vi "Precharge Control.vi"() -> ()   [LabVIEW 2014]
uses:
  Shutdown State Machine.lvsc/State.ctl
  Shutdown State Machine.lvsc/Inputs.ctl
  Shutdown State Machine.lvsc/StatechartState.ctl
  Shutdown State Machine.lvsc/CompanionDiagram.vi/2/SC Main.vi
  Shutdown State Machine.lvsc/CompanionDiagram.vi/2/Upd State.vi
  Shutdown State Machine.lvsc/CompanionDiagram.vi/2/Trans Graph0.vi
  Shutdown State Machine.lvsc/CompanionDiagram.vi/2/EnterGraphCore.vi
  <vilib>/FPGAPlugInAG/sbRIO-9626/niLvFpga_Open_sbRIO-9626.vi
  <vilib>/rvi/interface/common/dynamic/niFpgaDynamicAddResources.vi
  Global Data.vi
  <vilib>/Utility/error.llb/Error Cluster From Error Code.vi
  <vilib>/rvi/errors/niLvFpgaAdjustHostInterfaceError.vi
  Shutdown State Machine.lvsc/CompanionDiagram.vi
  <vilib>/FPGAPlugInAG/Dynamic/niLvFpga_Close_Dynamic.vi
  <vilib>/rvi/interface/nirviOpenFPGA/nirviOpenFPGA.xnode
  FPGA Bitfiles/FormulaElectric2_FPGATarget_FPGA_8a5J0mMac2U.lvbitx
  FPGA/Sensor Library/FPGA.vi
  Shutdown State Machine.lvsc/Trigger.ctl
  <vilib>/rvi/interface/nirviReadWriteControl/nirviReadWriteControl.xnode
  <vilib>/Statechart/Infrastructure/RTStatechart/RunTime SCN.xnode
  Shutdown State Machine.lvsc/Outputs.ctl
  AIR Status.ctl
  Shutdown State Machine.lvsc
  <vilib>/rvi/interface/nirviCloseFPGA/nirviCloseFPGA.xnode
  <vilib>/rvi/interface/Simulation/niFpgaSimulationCallBeginRW.vi
  NiFpgaLv.dll
panel:
  out "Shutdown State":T1
  in  "Precharge Time (msec)":u32=4000
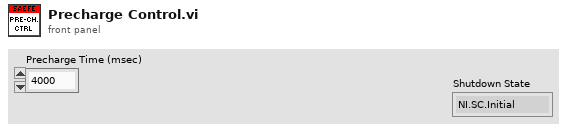
[diagram p1: front panel]
types:
  T1 = typedef "Shutdown State Machine.lvsc/State.ctl" = enum16{"NI.SC.Initial", "NI.SC.History", "NI.SC.ShallowHistory", "NI.SC.Terminal", "Precharge Finished/AIRs On", "Precharge", "TSMS Off"}
  T2 = typedef "Shutdown State Machine.lvsc/Inputs.ctl" = cluster{"TSMS Status In":bool, "Precharge Time":u32}
  T3 = typedef "Shutdown State Machine.lvsc/Outputs.ctl" = cluster{"Positive AIR Enable":bool, "AIR Status":T4, "Coolant Pump":bool}
  T4 = typedef "AIR Status.ctl" = enum16{"Off", "Precharge", "On"}
  T5 = typedef "Shutdown State Machine.lvsc/StatechartState.ctl" = T1[]
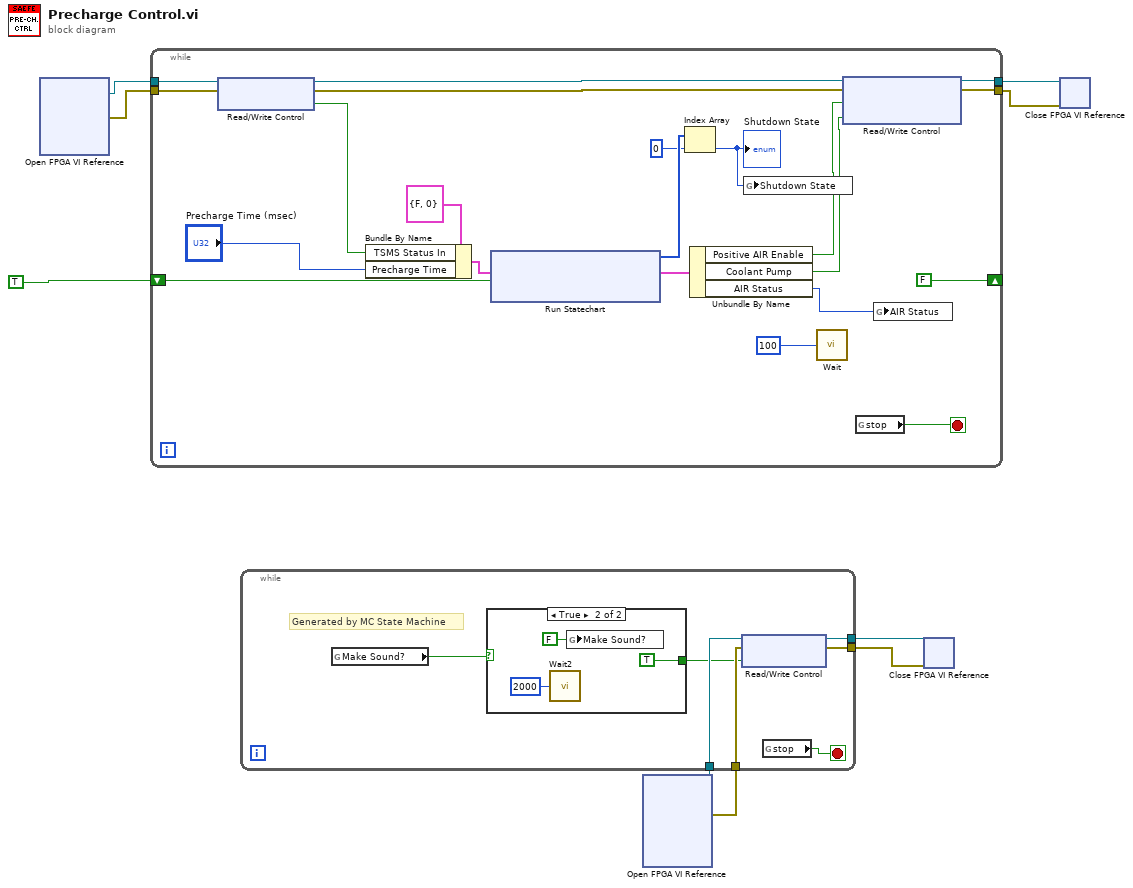
[diagram p0: block diagram]
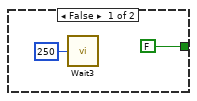
[diagram p2: hidden frame]
diagram:
  n1 = xnode "Open FPGA VI Reference"() -> ("FPGA VI Reference Out"=w9:refnum<k20>, "error out"=w6:errorcluster)  [unwired: 2 in]
  n2 = while {
    tunnel: w9 -> [w30]
    tunnel: [w25] -> w8
    tunnel: [w24] -> w7
    tunnel: w6 -> [w29]
    shift-right: [FALSE] -> _
    shift-left: TRUE -> [w23]
    stop <- w12 stop-if-true
    n3 = xnode "Read/Write Control"("FPGA VI Reference In"=w30, "error in"=w29) -> ("FPGA VI Reference Out"=w27:refnum<k20>, "error out"=w26:errorcluster, "TSMS In Status"=w19:bool)
    n4 = Bundle By Name(cluster=T2 {"TSMS Status In"=FALSE, "Precharge Time"=0} ("Inputs"), "TSMS Status In"=w19, "Precharge Time"="Precharge Time (msec)") -> (w20:T2)
    n5 = xnode "Run Statechart"("Init?"=w23, "Inputs"=w20) -> ("Outputs"=w17:T3, "Active States"=w16:T5)  [unwired: 1 in, 1 out]
    n6 = Index Array(array=w16, index=0) -> (element=w14:T1)
    "Shutdown State" <- w14
    n7 = Unbundle By Name(w17) -> ("Positive AIR Enable"=w11:bool, "Coolant Pump"=w10:bool, "AIR Status"=w13:T4)
    n8 = global write "Global Data.vi" "Shutdown State"(w14) -> ()
    n9 = call "Wait"("Count(mSec)"=u32 100) -> ()  [unwired: 1 out]
    n10 = xnode "Read/Write Control"("FPGA VI Reference In"=w27, "error in"=w26, "Positive AIR Enable"=w11, "Coolant Pump"=w10) -> ("FPGA VI Reference Out"=w25:refnum<k20>, "error out"=w24:errorcluster)
    n11 = global read "Global Data.vi" "stop"() -> (w12:bool)
    n12 = global write "Global Data.vi" "AIR Status"(w13) -> ()
  }
  n13 = xnode "Open FPGA VI Reference"() -> ("FPGA VI Reference Out"=w3:refnum<k20>, "error out"=w2:errorcluster)  [unwired: 2 in]
  n14 = while {
    tunnel: [w67] -> w5
    tunnel: [w66] -> w4
    tunnel: w3 -> [w65]
    tunnel: w2 -> [w64]
    stop <- w62 stop-if-true
    # "Generated by MC State Machine"
    n15 = global read "Global Data.vi" "Make Sound?"() -> (w68:bool)
    n16 = case shown="True" w68 {
      tunnel: [FALSE TRUE] -> w63
      frame False {
        n17 = call "Wait3"("Count(mSec)"=u32 250) -> ()  [unwired: 1 out]
      }
      frame True {
        n18 = call "Wait2"("Count(mSec)"=u32 2000) -> ()  [unwired: 1 out]
        n19 = global write "Global Data.vi" "Make Sound?"(FALSE ("Make Sound?")) -> ()
      }
    }
    n20 = xnode "Read/Write Control"("FPGA VI Reference In"=w65, "error in"=w64, "RTDS Enable"=w63) -> ("FPGA VI Reference Out"=w67:refnum<k20>, "error out"=w66:errorcluster)
    n21 = global read "Global Data.vi" "stop"() -> (w62:bool)
  }
  n22 = xnode "Close FPGA VI Reference"("FPGA VI Reference In"=w5, "error in"=w4) -> ()  [unwired: 1 out]
  n23 = xnode "Close FPGA VI Reference"("FPGA VI Reference In"=w8, "error in"=w7) -> ()  [unwired: 1 out]
